vi "Write PWM Ratio.vi"(8 "error in (no error)":errorcluster, 10 "PWM Ratio":dbl format="%.3g", 11 "Set Ratio Msg in":refnum<class "Set Ratio Msg.lvclass">) -> (0 "error out":errorcluster, 3 "Set Ratio Msg out":refnum<class "Set Ratio Msg.lvclass">)   [LabVIEW 2021, in "BNT_ULx.lvlib" / "Set Ratio Msg.lvclass"]
uses:
  Set Ratio Msg.lvclass
  Set Ratio Msg.lvclass/Set Ratio Msg.ctl
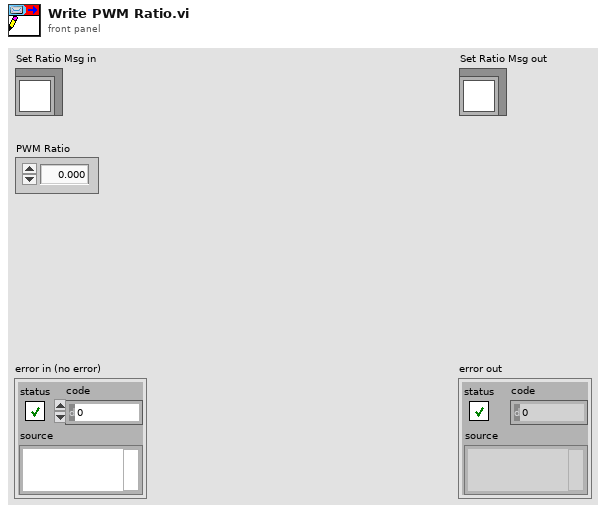
[diagram p1: front panel]
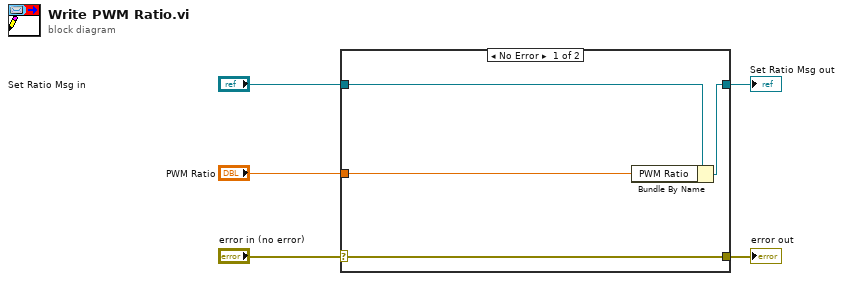
[diagram p0: block diagram]
diagram:
  n1 = case shown="No Error" "error in (no error)" {
    selector: "error in (no error)" -> [w9 w10]
    tunnel: [w9 w10] -> w4
    tunnel: [w7 w11] -> w2
    tunnel: "Set Ratio Msg in" -> [w8 w11]
    tunnel: "PWM Ratio" -> [w6 _]
    frame No Error {
      n2 = Bundle By Name(cluster=w8, "PWM Ratio"=w6) -> (w7:refnum<class "Set Ratio Msg.lvclass">)
    }
    frame Error {
    }
  }
  "error out" <- w4
  "Set Ratio Msg out" <- w2
